vi "Handle LAC Errors.vi"(8 "error in (no error)":errorcluster) -> ()   [LabVIEW 2018, in "Assert API Components.lvlib" / "Log Assert Core.lvlib"]
doc: "Logs any errors generated inside Log Assert Core to the specified debug method - either a log file or a debug UI"
uses:
  Log Assert Core.lvlib
  LAC Error Logger/LAC Error Logger.lvclass
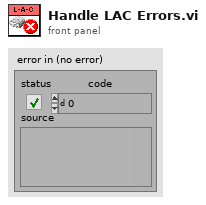
[diagram p1: front panel]
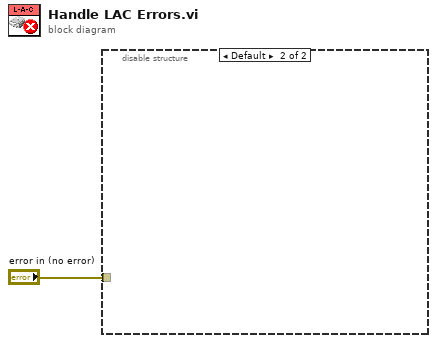
[diagram p0: block diagram]
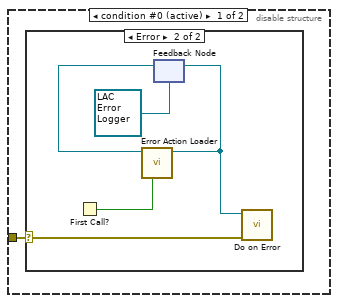
[diagram p2: hidden frame]
diagram:
  n1 = disable-structure shown="Default" {
    disable-tunnel: "error in (no error)" -> [w2 _]
    frame condition #0 (active) {
      n2 = case shown="Error" w2 {
        selector: w2 -> [_ w3]
        frame No Error {
        }
        frame Error {
          n3 = First Call?() -> (First Call?: T/F=w5:bool)
          n4 = feedback #1(refnum<class "LAC Error Logger.lvclass"> refnum ("Assert API Components.lvlib:Log Assert Core.lvlib:LAC Error Logger.lvclass")) -> (w7:refnum<class "LAC Error Logger.lvclass">)
          n5 = call "Error Action Loader.vi"("First Call?"=w5, "LAC Error Logger in"=w7) -> ("LAC Error Logger out"=w4:refnum<class "LAC Error Logger.lvclass">)  [unwired: 8 in, 1 out]
          n6 = feedback-in #1(w4) -> ()
          n7 = call-dynamic "Do on Error.vi"("error in (no error)"=w3, "LAC Error Logger in"=w4) -> ()  [unwired: 10 in]
        }
      }
    }
    frame condition #1 {
    }
  }
